vi "Error Global.vi"() -> ()   [LabVIEW 2021, in "CAN_Logic.lvclass"]
uses:
  CAN_Logic.lvclass
panel:
  in  "TX Timeout":errorcluster={"status"=TRUE, "code"=-8800, "source"="Timeout from the XNET Write.  Either the CAN network is unable to keep up with the amount of data being sent or there is no \"listener\" node on the network to ack the CAN message.  "}
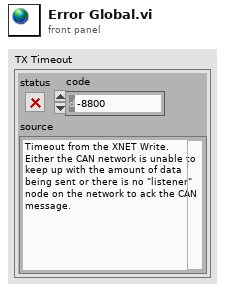
[diagram p1: front panel]
diagram:
